vi "UI--Initialize.vi"(8 "error in":errorcluster, 11 "Selector in":refnum<class "Selector.lvclass">) -> (0 "error out":errorcluster, 3 "Selector out":refnum<class "Selector.lvclass">)   [LabVIEW 2019, in "Selector.lvclass"]
uses:
  Selector.lvclass
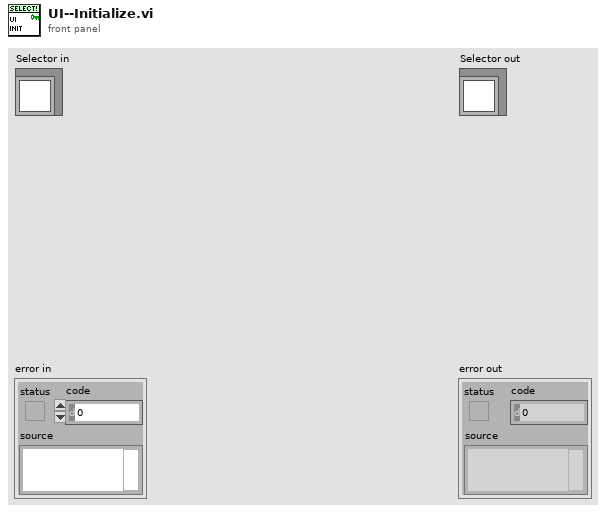
[diagram p1: front panel]
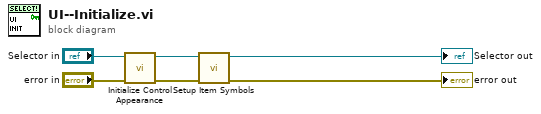
[diagram p0: block diagram]
diagram:
  n1 = call-dynamic "Initialize Control Appearance.vi"("error in (no error)"="error in", "Selector in"="Selector in") -> ("error out"=w5:errorcluster, "Selector out"=w6:refnum<class "Selector.lvclass">)  [unwired: 8 in]
  n2 = call-dynamic "Setup Item Symbols.vi"("error in (no error)"=w5, "Selector in"=w6) -> ("error out"=→"error out":errorcluster, "Selector out"=→"Selector out":refnum<class "Selector.lvclass">)  [unwired: 8 in]
